vi "Interpolate All Points (Distance).vi"(1 "Array in":cluster{"X":dbl, "Y":dbl}[](array[cluster])) -> (0 "Array out":cluster{"X":dbl, "Y":dbl}[](array[cluster]))   [LabVIEW 2013]
doc: "This VI uses the global variable Interpol. Dist. to interpolate points at given intervals in an array full of points."
uses:
  Global Variables.vi
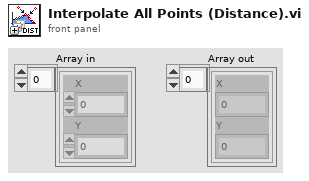
[diagram p1: front panel]
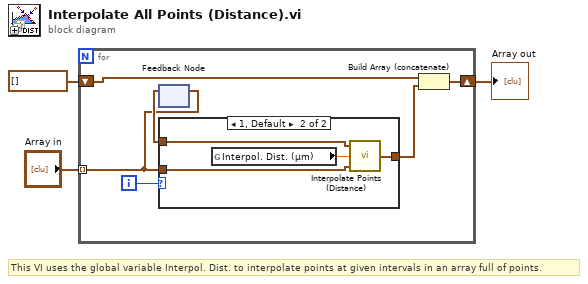
[diagram p0: block diagram]
diagram:
  # "This VI uses the global variable Interpol. Dist. to interpolate points at given intervals in an array full of points."
  n1 = for {
    shift-right: [w8] -> w1
    shift-left: cluster{"X":dbl, "Y":dbl}[] [] -> [w7]
    tunnel: "Array in" -> [w5] mode=indexing
    i -> [w4]
    n2 = feedback-in #1(w5) -> ()
    n3 = feedback #1() -> (w6:cluster{"X":dbl, "Y":dbl})  [unwired: 1 in]
    n4 = case shown="1, Default" w4 {
      tunnel: [_ w13] -> w9
      tunnel: w6 -> [_ w10]
      tunnel: w5 -> [_ w11]
      frame 0 {
      }
      frame 1, Default {
        n5 = global read "Global Variables.vi" "Interpol. Dist. (µm)"() -> (w12:dbl)
        n6 = call "Interpolate Points (Distance).vi"("End Point"=w11, "Distance between Points"=w12, "Start Point"=w10) -> ("Output Point Array"=w13:cluster{"X":dbl, "Y":dbl}[])
      }
    }
    n7 = Build Array (concatenate)(w7, w9) -> (w8:cluster{"X":dbl, "Y":dbl}[])
  }
  "Array out" <- w1
